vi "CB Target.vi"(0 "IVI Refnum in":refnum<k15>, 1 "Write Targets":dbl[][](array[numeric]), 2 "Check First?":bool, 3 "CB offset":i32, 4 "CB size":i32, 5 "error in (no error)":errorcluster, 6 "CB write outfile":path, 7 "i":i32, 10 "MLC WLV":dbl[][](array[numeric]), 11 "CB type":u16, 12 "Write Algorithm":u16) -> (14 "IVI Refnum out":refnum<k15>, 15 "final current (A)":dbl, 17 "final resistance (ohm)":dbl, 19 "error out":errorcluster)   [LabVIEW 2018]
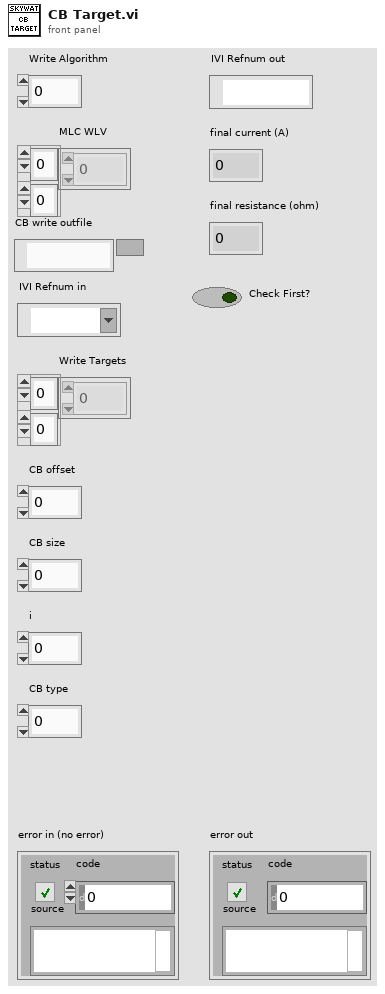
[diagram p1: front panel]
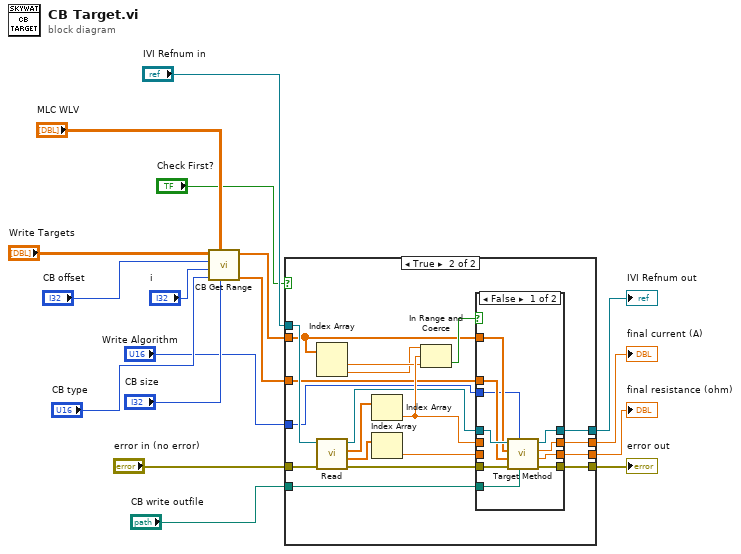
[diagram p0: block diagram]
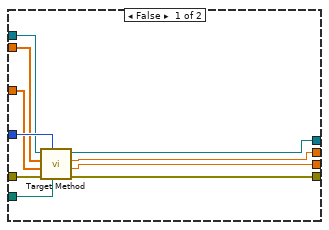
[diagram p2: hidden frame]
diagram:
  n1 = call "CB Get Range.vi"("CB size"="CB size", "Algo Params"="MLC WLV", "CB type"="CB type", "i"="i", "CB offset"="CB offset", "Write Targets"="Write Targets") -> ("Algo Param"=w2:dbl[], "Write Target"=w3:dbl[])  [unwired: 4 in]
  n2 = case shown="True" "Check First?" {
    tunnel: "CB write outfile" -> [w27 w32]
    tunnel: "Write Algorithm" -> [w26 w31]
    tunnel: [w25 w40] -> w9
    tunnel: [w24 w39] -> w8
    tunnel: [w23 w35] -> w7
    tunnel: "error in (no error)" -> [w22 w46]
    tunnel: [w21 w34] -> w5
    tunnel: "IVI Refnum in" -> [w20 w45]
    tunnel: w3 -> [w19 w30]
    tunnel: w2 -> [w18 w33]
    frame False {
      n3 = call "Target Method.vi"("Target outfile"=w27, "Algorithm"=w26, "error in (no error)"=w22, "Algo Param"=w18, "Write Target"=w19, "IVI Refnum in"=w20) -> ("error out"=w23:errorcluster, "final resistance (ohm)"=w24:dbl, "final current (A)"=w25:dbl, "IVI Refnum out"=w21:refnum<k15>)  [unwired: 2 in]
    }
    frame True {
      n4 = Index Array(array=w30) -> (element #1=w29:dbl, element #2=w28:dbl)  [unwired: 2 in]
      n5 = call "Read.vi"("error in (no error)"=w46, "instrument handle"=w45) -> ("error out"=w36:errorcluster, "currents (A)"=w43:dbl[], "resistances (ohm)"=w44:dbl[], "instrument handle out"=w37:refnum<k15>)  [unwired: 6 in]
      n6 = Index Array(array=w44) -> (element=w38:dbl)  [unwired: 1 in]
      n7 = Index Array(array=w43) -> (element=w41:dbl)  [unwired: 1 in]
      n8 = In Range and Coerce(upper limit=w28, x=w38, lower limit=w29) -> (In Range?=w42:bool)  [unwired: 1 out]
      n9 = case shown="False" w42 {
        tunnel: w41 -> [_ w60]
        tunnel: [w51 w60] -> w40
        tunnel: [w52 w59] -> w39
        tunnel: w38 -> [_ w59]
        tunnel: w37 -> [w56 w57]
        tunnel: w36 -> [w55 w58]
        tunnel: [w54 w58] -> w35
        tunnel: [w53 w57] -> w34
        tunnel: w30 -> [w50 _]
        tunnel: w33 -> [w49 _]
        tunnel: w32 -> [w48 _]
        tunnel: w31 -> [w47 _]
        frame False {
          n10 = call "Target Method.vi"("Target outfile"=w48, "Algorithm"=w47, "error in (no error)"=w55, "Algo Param"=w49, "Write Target"=w50, "IVI Refnum in"=w56) -> ("error out"=w54:errorcluster, "final resistance (ohm)"=w52:dbl, "final current (A)"=w51:dbl, "IVI Refnum out"=w53:refnum<k15>)  [unwired: 2 in]
        }
        frame True {
        }
      }
    }
  }
  "final current (A)" <- w9
  "final resistance (ohm)" <- w8
  "error out" <- w7
  "IVI Refnum out" <- w5
